vi "Run_Core.vi"(0 "Message Popup in":refnum<class "Array Functions.lvclass">, 11 "error in (no error)":errorcluster) -> (4 "Message Popup out":refnum<class "Array Functions.lvclass">, 6 "Return":variant, 15 "error out":errorcluster)   [LabVIEW 2016, in "Array Functions.lvclass"]
uses:
  Array Functions.lvclass
  Array Functions.lvclass/Array Functions.ctl
  data types/Variant to Data/Var to Numeric.vi
  data types/Variant to Data/Var to String.vi
  data types/Variant to Data/Var to Boolean.vi
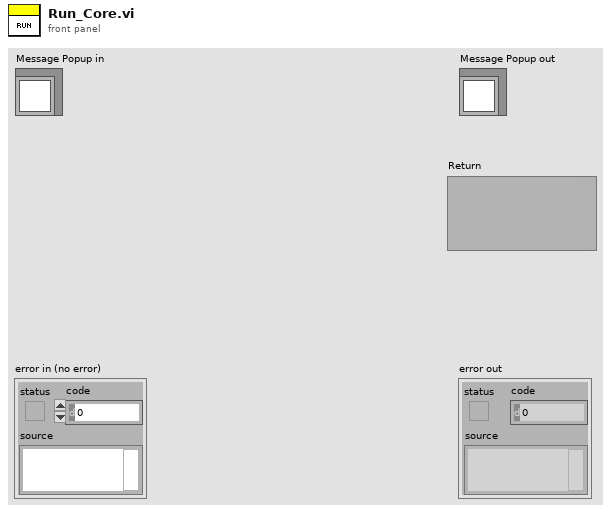
[diagram p1: front panel]
types:
  T1 = typedef "Array Functions.lvclass/Function List.ctl" = enum16{"Array Size", "Index Array", "Replace Subset", "Insert Into Array", "Delete From Array", "Initialize Array", "Build Array", "Array Subset", "Max in Array", "Min in Array", "Sort 1D Array", "Search 1D Aray", "Reverse 1D Array"}
  T2 = typedef "Datatype.ctl" = enum16{"Null", "Numeric", "String", "Bool", "Numeric 1D", "String 1D", "Bool 1D", "Numeric 2D", "String 2D", "Bool 2D", "Variant"}
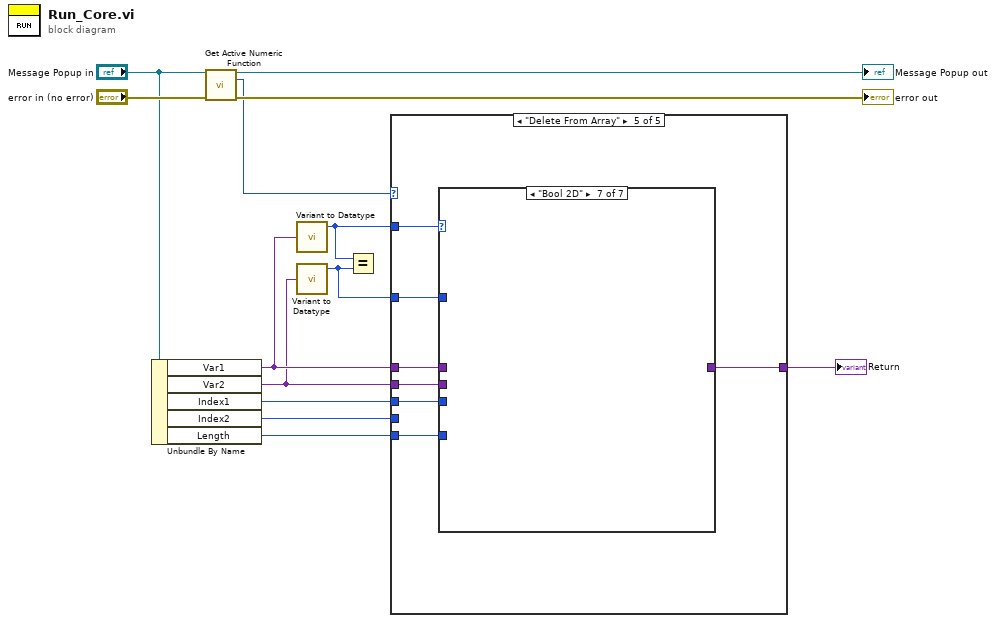
[diagram p0: block diagram]
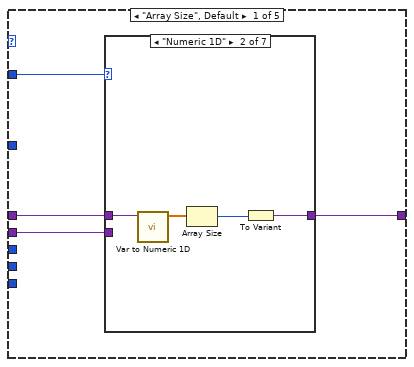
[diagram p2: hidden frame]
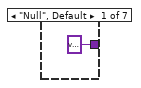
[diagram p3: hidden frame]
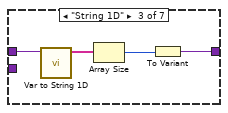
[diagram p4: hidden frame]
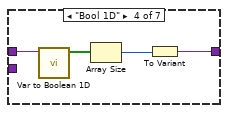
[diagram p5: hidden frame]
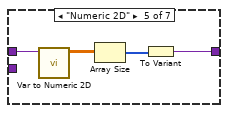
[diagram p6: hidden frame]
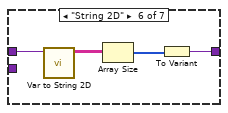
[diagram p7: hidden frame]
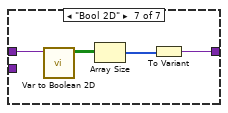
[diagram p8: hidden frame]
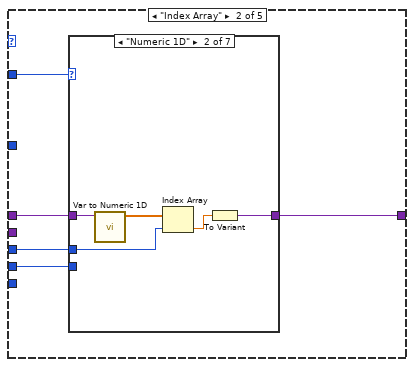
[diagram p9: hidden frame]
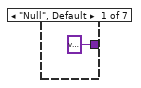
[diagram p10: hidden frame]
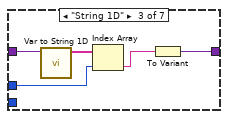
[diagram p11: hidden frame]
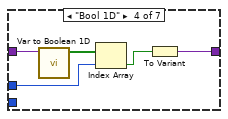
[diagram p12: hidden frame]
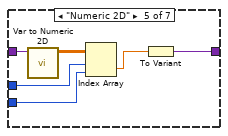
[diagram p13: hidden frame]
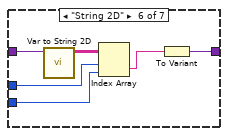
[diagram p14: hidden frame]
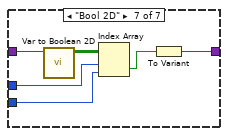
[diagram p15: hidden frame]
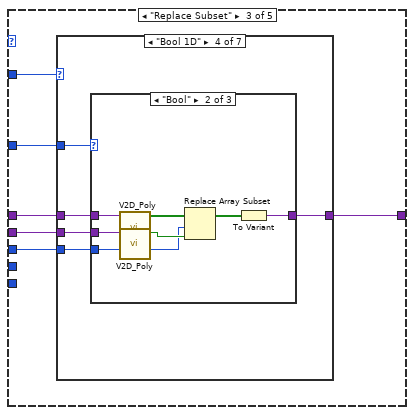
[diagram p16: hidden frame]
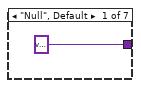
[diagram p17: hidden frame]
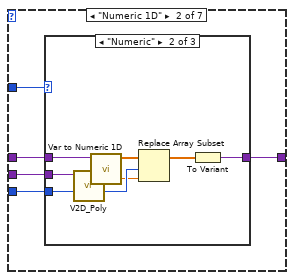
[diagram p18: hidden frame]
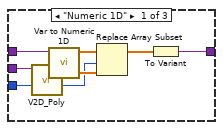
[diagram p19: hidden frame]
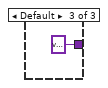
[diagram p20: hidden frame]
diagram:
  n1 = Unbundle By Name("Message Popup in") -> ("Var1"=w8:variant, "Var2"=w3:variant, "Index1"=w5:i32, "Index2"=w4:i32, "Length"=w1:i32)
  n2 = call "Get Active Numeric Function.vi"("Numeric Functions in"="Message Popup in", "error in (no error)"="error in (no error)") -> ("Numeric Functions out"=→"Message Popup out":refnum<class "Array Functions.lvclass">, "Function"=w9:T1, "error out"=→"error out":errorcluster)  [unwired: 11 in]
  n3 = call "Variant to Datatype.vi"("Variant"=w8) -> ("Datatype"=w7:T2)  [unwired: 2 in, 2 out]
  n4 = call "Variant to Datatype.vi"("Variant"=w3) -> ("Datatype"=w2:T2)  [unwired: 2 in, 2 out]
  n5 = Equal?(x=w7, y=w2) -> ()  [unwired: 1 out]
  n6 = case shown="\"Delete From Array\"" w9 {
    tunnel: w8 -> [w17 w47 w87 w154 w222]
    tunnel: w3 -> [w16 _ w84 w151 w219]
    tunnel: w7 -> [w15 w44 w82 w149 w217]
    tunnel: [w14 w46 w86 w153 w221] -> w6
    tunnel: w5 -> [_ w45 w83 w150 w218]
    tunnel: w4 -> [_ w43 _ _ _]
    tunnel: w2 -> [_ _ w85 w152 w220]
    tunnel: w1 -> [_ _ _ _ w216]
    frame "Array Size", Default {
      n7 = case shown="\"Numeric 1D\"" w15 {
        tunnel: w17 -> [_ w22 w26 w30 w34 w38 w42]
        tunnel: w16 -> [_ _ _ _ _ _ _]
        tunnel: [variant ("Variant") w19 w23 w27 w31 w35 w39] -> w14
        frame "Null", Default {
        }
        frame "Numeric 1D" {
          n8 = call "Var to Numeric 1D.vi"("Variant"=w22) -> ("Numeric Array"=w21:dbl[])  [unwired: 10 in]
          n9 = Array Size(array=w21) -> (size(s)=w20:i32)
          n10 = To Variant(anything=w20) -> (Variant=w19:variant)
        }
        frame "String 1D" {
          n11 = call "Var to String 1D.vi"("Variant"=w26) -> ("String 1D"=w24:string[])  [unwired: 10 in]
          n12 = Array Size(array=w24) -> (size(s)=w25:i32)
          n13 = To Variant(anything=w25) -> (Variant=w23:variant)
        }
        frame "Bool 1D" {
          n14 = call "Var to Boolean 1D.vi"("Variant"=w30) -> ("Bool 1D"=w28:bool[])  [unwired: 10 in]
          n15 = Array Size(array=w28) -> (size(s)=w29:i32)
          n16 = To Variant(anything=w29) -> (Variant=w27:variant)
        }
        frame "Numeric 2D" {
          n17 = call "Var to Numeric 2D.vi"("Variant"=w34) -> ("Numeric Array"=w32:dbl[][])  [unwired: 10 in]
          n18 = Array Size(array=w32) -> (size(s)=w33:i32[])
          n19 = To Variant(anything=w33) -> (Variant=w31:variant)
        }
        frame "String 2D" {
          n20 = call "Var to String 2D.vi"("Variant"=w38) -> ("String 2D"=w36:string[][])  [unwired: 10 in]
          n21 = Array Size(array=w36) -> (size(s)=w37:i32[])
          n22 = To Variant(anything=w37) -> (Variant=w35:variant)
        }
        frame "Bool 2D" {
          n23 = call "Var to Boolean 2D.vi"("Variant"=w42) -> ("Bool 2D"=w40:bool[][])  [unwired: 10 in]
          n24 = Array Size(array=w40) -> (size(s)=w41:i32[])
          n25 = To Variant(anything=w41) -> (Variant=w39:variant)
        }
      }
    }
    frame "Index Array" {
      n26 = case shown="\"Numeric 1D\"" w44 {
        tunnel: w47 -> [_ w53 w58 w63 w69 w75 w81]
        tunnel: [variant ("Variant") w52 w57 w62 w68 w74 w80] -> w46
        tunnel: w45 -> [_ w50 w54 w59 w65 w71 w77]
        tunnel: w43 -> [_ _ _ _ w64 w70 w76]
        frame "Null", Default {
        }
        frame "Numeric 1D" {
          n27 = call "Var to Numeric 1D.vi"("Variant"=w53) -> ("Numeric Array"=w51:dbl[])  [unwired: 10 in]
          n28 = Index Array(array=w51, index=w50) -> (element=w49:dbl)
          n29 = To Variant(anything=w49) -> (Variant=w52:variant)
        }
        frame "String 1D" {
          n30 = call "Var to String 1D.vi"("Variant"=w58) -> ("String 1D"=w56:string[])  [unwired: 10 in]
          n31 = Index Array(array=w56, index=w54) -> (element=w55:string)
          n32 = To Variant(anything=w55) -> (Variant=w57:variant)
        }
        frame "Bool 1D" {
          n33 = call "Var to Boolean 1D.vi"("Variant"=w63) -> ("Bool 1D"=w61:bool[])  [unwired: 10 in]
          n34 = Index Array(array=w61, index=w59) -> (element=w60:bool)
          n35 = To Variant(anything=w60) -> (Variant=w62:variant)
        }
        frame "Numeric 2D" {
          n36 = call "Var to Numeric 2D.vi"("Variant"=w69) -> ("Numeric Array"=w67:dbl[][])  [unwired: 10 in]
          n37 = Index Array(array=w67, index (row)=w65, index (col)=w64) -> (element=w66:dbl)
          n38 = To Variant(anything=w66) -> (Variant=w68:variant)
        }
        frame "String 2D" {
          n39 = call "Var to String 2D.vi"("Variant"=w75) -> ("String 2D"=w73:string[][])  [unwired: 10 in]
          n40 = Index Array(array=w73, index (row)=w71, index (col)=w70) -> (element=w72:string)
          n41 = To Variant(anything=w72) -> (Variant=w74:variant)
        }
        frame "Bool 2D" {
          n42 = call "Var to Boolean 2D.vi"("Variant"=w81) -> ("Bool 2D"=w79:bool[][])  [unwired: 10 in]
          n43 = Index Array(array=w79, index (row)=w77, index (col)=w76) -> (element=w78:bool)
          n44 = To Variant(anything=w78) -> (Variant=w80:variant)
        }
      }
    }
    frame "Replace Subset" {
      n45 = case shown="\"Bool 1D\"" w82 {
        tunnel: w87 -> [_ w93 w113 w133 _ _ _]
        tunnel: [variant ("Variant") w92 w109 w130 _ _ _] -> w86
        tunnel: w83 -> [_ w89 w110 w131 _ _ _]
        tunnel: w85 -> [_ w91 w112 w129 _ _ _]
        tunnel: w84 -> [_ w90 w111 w132 _ _ _]
        frame "Null", Default {
        }
        frame "Numeric 1D" {
          n46 = case shown="\"Numeric\"" w91 {
            tunnel: w93 -> [w97 w107 _]
            tunnel: [w96 w106 variant ("Variant")] -> w92
            tunnel: w90 -> [w95 w103 _]
            tunnel: w89 -> [w94 w102 _]
            frame "Numeric 1D" {
              n47 = call-poly "V2D_Poly.vi"("Variant"=w95) -> ("Numeric Array"=w98:dbl[])  [unwired: 10 in]
              n48 = call "Var to Numeric 1D.vi"("Variant"=w97) -> ("Numeric Array"=w100:dbl[])  [unwired: 10 in]
              n49 = Replace Array Subset(array=w100, new element=w98, index=w94) -> (w99:dbl[])
              n50 = To Variant(anything=w99) -> (Variant=w96:variant)
            }
            frame "Numeric" {
              n51 = call-poly "V2D_Poly.vi"("Variant"=w103) -> ("Numeric"=w101:dbl)  [unwired: 10 in]
              n52 = call "Var to Numeric 1D.vi"("Variant"=w107) -> ("Numeric Array"=w105:dbl[])  [unwired: 10 in]
              n53 = Replace Array Subset(array=w105, new element=w101, index=w102) -> (w104:dbl[])
              n54 = To Variant(anything=w104) -> (Variant=w106:variant)
            }
            frame Default {
            }
          }
        }
        frame "String 1D" {
          n55 = case shown="\"String\"" w112 {
            tunnel: w113 -> [w117 w124 _]
            tunnel: [w118 w127 variant ("Variant")] -> w109
            tunnel: w111 -> [w115 w122 _]
            tunnel: w110 -> [w114 w121 _]
            frame "String 1D" {
              n56 = call-poly "V2D_Poly.vi"("Variant"=w117) -> ("String 1D"=w116:string[])  [unwired: 10 in]
              n57 = call-poly "V2D_Poly.vi"("Variant"=w115) -> ("String 1D"=w119:string[])  [unwired: 10 in]
              n58 = Replace Array Subset(array=w116, new element=w119, index=w114) -> (w120:string[])
              n59 = To Variant(anything=w120) -> (Variant=w118:variant)
            }
            frame "String" {
              n60 = call-poly "V2D_Poly.vi"("Variant"=w124) -> ("String 1D"=w123:string[])  [unwired: 10 in]
              n61 = call-poly "V2D_Poly.vi"("Variant"=w122) -> ("String"=w125:string)  [unwired: 10 in]
              n62 = Replace Array Subset(array=w123, new element=w125, index=w121) -> (w126:string[])
              n63 = To Variant(anything=w126) -> (Variant=w127:variant)
            }
            frame Default {
            }
          }
        }
        frame "Bool 1D" {
          n64 = case shown="\"Bool\"" w129 {
            tunnel: w133 -> [w137 w144 _]
            tunnel: [w138 w147 variant ("Variant")] -> w130
            tunnel: w132 -> [w135 w142 _]
            tunnel: w131 -> [w134 w141 _]
            frame "Bool 1D" {
              n65 = call-poly "V2D_Poly.vi"("Variant"=w137) -> ("Bool 1D"=w136:bool[])  [unwired: 10 in]
              n66 = call-poly "V2D_Poly.vi"("Variant"=w135) -> ("Bool 1D"=w139:bool[])  [unwired: 10 in]
              n67 = Replace Array Subset(array=w136, new element=w139, index=w134) -> (w140:bool[])
              n68 = To Variant(anything=w140) -> (Variant=w138:variant)
            }
            frame "Bool" {
              n69 = call-poly "V2D_Poly.vi"("Variant"=w144) -> ("Bool 1D"=w143:bool[])  [unwired: 10 in]
              n70 = call-poly "V2D_Poly.vi"("Variant"=w142) -> ("Boolean"=w145:bool)  [unwired: 10 in]
              n71 = Replace Array Subset(array=w143, new element=w145, index=w141) -> (w146:bool[])
              n72 = To Variant(anything=w146) -> (Variant=w147:variant)
            }
            frame Default {
            }
          }
        }
        frame "Numeric 2D" {
        }
        frame "String 2D" {
        }
        frame "Bool 2D" {
        }
      }
    }
    frame "Insert Into Array" {
      n73 = case shown="\"Numeric 2D\"" w149 {
        tunnel: w154 -> [_ w160 w180 w200 _ _ _]
        tunnel: [variant ("Variant") w159 w176 w197 _ _ _] -> w153
        tunnel: w150 -> [_ w156 w177 w198 _ _ _]
        tunnel: w152 -> [_ w158 w179 w196 _ _ _]
        tunnel: w151 -> [_ w157 w178 w199 _ _ _]
        frame "Null", Default {
        }
        frame "Numeric 1D" {
          n74 = case shown="\"Numeric\"" w158 {
            tunnel: w160 -> [w164 w174 _]
            tunnel: [w163 w173 variant ("Variant")] -> w159
            tunnel: w157 -> [w162 w170 _]
            tunnel: w156 -> [w161 w169 _]
            frame "Numeric 1D" {
              n75 = call-poly "V2D_Poly.vi"("Variant"=w162) -> ("Numeric Array"=w165:dbl[])  [unwired: 10 in]
              n76 = call "Var to Numeric 1D.vi"("Variant"=w164) -> ("Numeric Array"=w167:dbl[])  [unwired: 10 in]
              n77 = Insert Into Array(array=w167, index=w161, new element=w165) -> (w166:dbl[])
              n78 = To Variant(anything=w166) -> (Variant=w163:variant)
            }
            frame "Numeric" {
              n79 = call-poly "V2D_Poly.vi"("Variant"=w170) -> ("Numeric"=w168:dbl)  [unwired: 10 in]
              n80 = call "Var to Numeric 1D.vi"("Variant"=w174) -> ("Numeric Array"=w172:dbl[])  [unwired: 10 in]
              n81 = Insert Into Array(array=w172, index=w169, new element=w168) -> (w171:dbl[])
              n82 = To Variant(anything=w171) -> (Variant=w173:variant)
            }
            frame Default {
            }
          }
        }
        frame "String 1D" {
          n83 = case shown="Default" w179 {
            tunnel: w180 -> [w184 w191 _]
            tunnel: [w185 w194 variant ("Variant")] -> w176
            tunnel: w178 -> [w182 w189 _]
            tunnel: w177 -> [w181 w188 _]
            frame "String 1D" {
              n84 = call-poly "V2D_Poly.vi"("Variant"=w184) -> ("String 1D"=w183:string[])  [unwired: 10 in]
              n85 = call-poly "V2D_Poly.vi"("Variant"=w182) -> ("String 1D"=w186:string[])  [unwired: 10 in]
              n86 = Insert Into Array(array=w183, index=w181, new element=w186) -> (w187:string[])
              n87 = To Variant(anything=w187) -> (Variant=w185:variant)
            }
            frame "String" {
              n88 = call-poly "V2D_Poly.vi"("Variant"=w191) -> ("String 1D"=w190:string[])  [unwired: 10 in]
              n89 = call-poly "V2D_Poly.vi"("Variant"=w189) -> ("String"=w192:string)  [unwired: 10 in]
              n90 = Insert Into Array(array=w190, index=w188, new element=w192) -> (w193:string[])
              n91 = To Variant(anything=w193) -> (Variant=w194:variant)
            }
            frame Default {
            }
          }
        }
        frame "Bool 1D" {
          n92 = case shown="\"Bool\"" w196 {
            tunnel: w200 -> [w204 w211 _]
            tunnel: [w205 w214 variant ("Variant")] -> w197
            tunnel: w199 -> [w202 w209 _]
            tunnel: w198 -> [w201 w208 _]
            frame "Bool 1D" {
              n93 = call-poly "V2D_Poly.vi"("Variant"=w204) -> ("Bool 1D"=w203:bool[])  [unwired: 10 in]
              n94 = call-poly "V2D_Poly.vi"("Variant"=w202) -> ("Bool 1D"=w206:bool[])  [unwired: 10 in]
              n95 = Insert Into Array(array=w203, index=w201, new element=w206) -> (w207:bool[])
              n96 = To Variant(anything=w207) -> (Variant=w205:variant)
            }
            frame "Bool" {
              n97 = call-poly "V2D_Poly.vi"("Variant"=w211) -> ("Bool 1D"=w210:bool[])  [unwired: 10 in]
              n98 = call-poly "V2D_Poly.vi"("Variant"=w209) -> ("Boolean"=w212:bool)  [unwired: 10 in]
              n99 = Insert Into Array(array=w210, index=w208, new element=w212) -> (w213:bool[])
              n100 = To Variant(anything=w213) -> (Variant=w214:variant)
            }
            frame Default {
            }
          }
        }
        frame "Numeric 2D" {
        }
        frame "String 2D" {
        }
        frame "Bool 2D" {
        }
      }
    }
    frame "Delete From Array" {
      n101 = case shown="\"Bool 2D\"" w217 {
        tunnel: w222 -> [_ w229 w235 w241 _ _ _]
        tunnel: [variant ("Variant") w228 w234 w240 _ _ _] -> w221
        tunnel: w218 -> [_ w225 w231 w237 _ _ _]
        tunnel: w220 -> [_ _ _ _ _ _ _]
        tunnel: w219 -> [_ _ _ _ _ _ _]
        tunnel: w216 -> [_ w224 w230 w236 _ _ _]
        frame "Null", Default {
        }
        frame "Numeric 1D" {
          n102 = call "Var to Numeric 1D.vi"("Variant"=w229) -> ("Numeric Array"=w227:dbl[])  [unwired: 10 in]
          n103 = Delete From Array(array=w227, length=w224, index=w225) -> (array with subset deleted=w226:dbl[])  [unwired: 1 out]
          n104 = To Variant(anything=w226) -> (Variant=w228:variant)
        }
        frame "String 1D" {
          n105 = call-poly "V2D_Poly.vi"("Variant"=w235) -> ("String 1D"=w232:string[])  [unwired: 10 in]
          n106 = Delete From Array(array=w232, length=w230, index=w231) -> (array with subset deleted=w233:string[])  [unwired: 1 out]
          n107 = To Variant(anything=w233) -> (Variant=w234:variant)
        }
        frame "Bool 1D" {
          n108 = call-poly "V2D_Poly.vi"("Variant"=w241) -> ("Bool 1D"=w238:bool[])  [unwired: 10 in]
          n109 = Delete From Array(array=w238, length=w236, index=w237) -> (array with subset deleted=w239:bool[])  [unwired: 1 out]
          n110 = To Variant(anything=w239) -> (Variant=w240:variant)
        }
        frame "Numeric 2D" {
        }
        frame "String 2D" {
        }
        frame "Bool 2D" {
        }
      }
    }
  }
  "Return" <- w6
